vi "SetService.vi"(4 "Properties in Service":string[](array[string]), 6 "Service Name":string, 7 "Properties":string[][](array[string]), 8 "error in":errorcluster, 9 "appKey":string, 10 "uri beginning":string, 11 "client handle":T1) -> (0 "error out":errorcluster, 1 "appKey out":string, 2 "uri beginning out":string, 3 "client handle out":T1, 5 "body":string)   [LabVIEW 2015]
uses:
  <vilib>/httpClient/ClientHandle.ctl
  <vilib>/httpClient/POSTBuffer.vi
  <vilib>/httpClient/LabVIEWHTTPClient.lvlib
panel:
  out "final url":string
  # "http://52.202.159.58:80/Thingworx/Things/GenericEdge/Services/UpdateValues?appKey=0aae8b5f-871a-4973-bdf2-199fabb27dcb&method=post&x-thingworx-session=true<&Photocell=11.00&Potentiometer=9.00&Temperature=0.00&Button=true>\n\nhttp://52.202.159.58:80/Thingworx/Things/GenericEdge/Services/UpdateValues?appKey=0aae8b5f-871a-4973-bdf2-199fabb27dcb&method=post&x-thingworx-session=true<&Temperature=2&Photocell=7&Button=0&Potentiometer=10>"
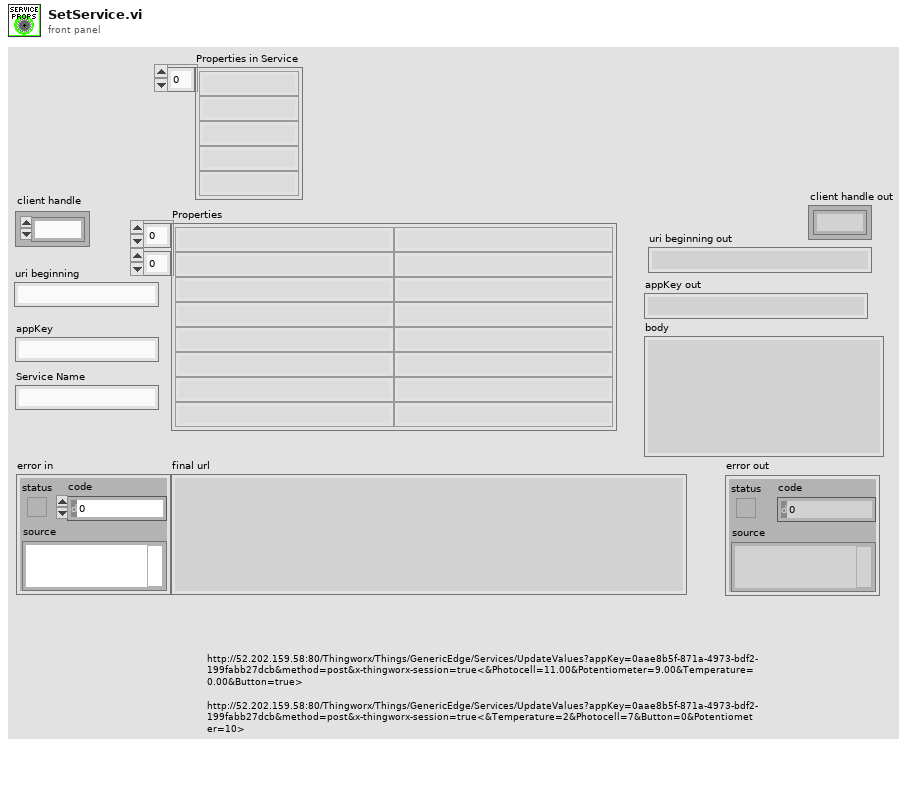
[diagram p1: front panel]
types:
  T1 = typedef "LabVIEWHTTPClient.lvlib/ClientHandle.ctl" = refnum<k1>
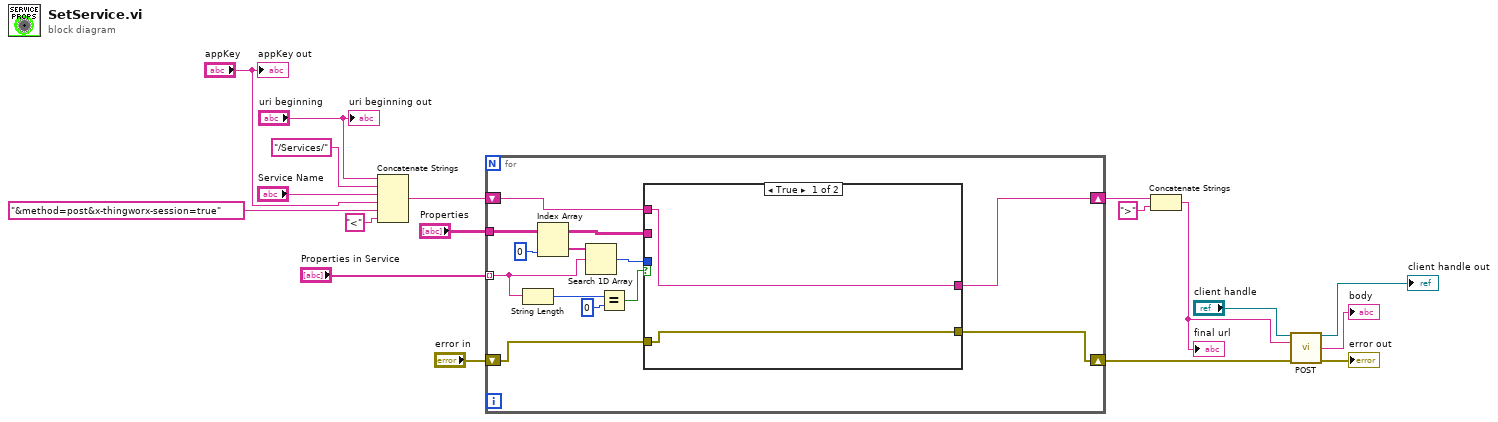
[diagram p0: block diagram]
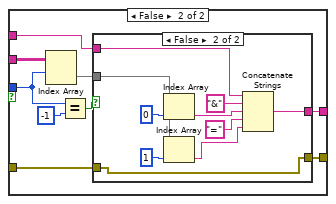
[diagram p2: hidden frame]
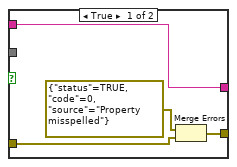
[diagram p3: hidden frame]
diagram:
  n1 = Concatenate Strings("uri beginning", "/Services/" ("string"), "Service Name", "appKey", "&method=post&x-thingworx-session=true" ("string"), "<" ("string")) -> (w9:string)
  n2 = for {
    tunnel: "Properties" -> [w28]
    shift-right: [w29] -> w8
    shift-left: w9 -> [w30]
    tunnel: "Properties in Service" -> [w24] mode=indexing
    shift-right: [w19] -> w1
    shift-left: "error in" -> [w20]
    n3 = String Length(string=w24) -> (length=w23:i32)
    n4 = Index Array(array=w28, index (col)=0 ("disabled index (col)")) -> (element=w26:string[])  [unwired: 1 in]
    n5 = Search 1D Array(1D array=w26, element=w24) -> (index of element=w25:i32)  [unwired: 1 in]
    n6 = Equal?(x=w23, y=0) -> (x = y?=w21:bool)
    n7 = case shown="True" w21 {
      tunnel: w30 -> [w32 w41]
      tunnel: [w32 w40] -> w29
      tunnel: w28 -> [_ w38]
      tunnel: w25 -> [_ w37]
      tunnel: w20 -> [w31 w34]
      tunnel: [w31 w33] -> w19
      frame True {
      }
      frame False {
        n8 = Index Array(array=w38, index (row)=w37) -> (element=w36:string[])  [unwired: 1 in]
        n9 = Equal?(x=w37, y=-1) -> (x = y?=w35:bool)
        n10 = case shown="False" w35 {
          tunnel: w41 -> [w42 w54]
          tunnel: [w42 w52] -> w40
          tunnel: w36 -> [_ w51]
          tunnel: w34 -> [w45 w46]
          tunnel: [w43 w46] -> w33
          frame True {
            n11 = Merge Errors(errorcluster {"status"=TRUE, "code"=0, "source"="Property misspelled"} ("error in"), w45) -> (w43:errorcluster)
          }
          frame False {
            n12 = Index Array(array=w51, index=0) -> (element=w48:string)
            n13 = Index Array(array=w51, index=1) -> (element=w50:string)
            n14 = Concatenate Strings(w54, "&" ("string"), w48, "=" ("string"), w50) -> (w52:string)
          }
        }
      }
    }
  }
  n15 = Concatenate Strings(w8, ">" ("string")) -> (w7:string)
  "final url" <- w7
  n16 = call-poly <vilib>:"POST.vi"("client handle"="client handle", "url"=w7, "error in (no error)"=w1) -> ("client handle out"=→"client handle out":T1, "body"=→"body":string, "error out"=→"error out":errorcluster)  [unwired: 9 in, 1 out]
  "uri beginning out" <- "uri beginning"
  "appKey out" <- "appKey"
